vi "Monitor for Stop.vi"(7 "timeout":i32=200, 8 "error in (no error)":errorcluster, 9 "Mixed Mode Commands In":refnum<queue>, 11 "MM Button Events In":refnum<notifier>) -> (0 "error out":errorcluster, 1 "Mixed Mode Commands Out":refnum<queue>, 2 "Stop Requests":T1, 3 "Button Events Out":refnum<notifier>)   [LabVIEW 2009]
uses:
  MixedMode/Messages/Mixed Mode Button Events Message.ctl
  MixedMode/Messages/Mixed Mode Button Events.ctl
  Mixed Mode Widget Button States.ctl
  MixedMode/Messages/Mixed Mode Command.ctl
  MixedMode/Mixed Mode Command Action.ctl
  MixedMode/Ramp Time Tuple.ctl
  MixedMode/Target Data.ctl
  Stop Requests.ctl
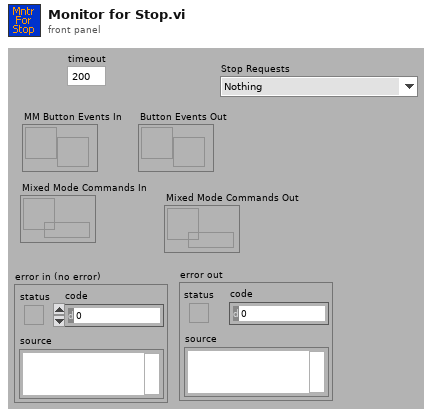
[diagram p1: front panel]
types:
  T1 = typedef "Stop Requests.ctl" = enum16{"Nothing", "Stop Requested", "Abort Requested"}
  T2 = typedef "Mixed Mode Command.ctl" = cluster{"Command":T3, "Ramp Times":cluster{"Initial":T4, "Iterative":T4}, "LBCB1":T5, "LBCB2":T5}
  T3 = typedef "Mixed Mode Command Action.ctl" = enum16{"Start Command", "Stop", "Exit", "No Op", "Start Acquisition", "Measure Initial Position"}
  T4 = typedef "Ramp Time Tuple.ctl" = cluster{"Ramp":dbl, "Stab":dbl, "Hold":dbl}
  T5 = typedef "Target Data.ctl" = cluster{"Displacements":dbl[], "Command Type":enum16{"<None>", "Displacement", "Force"}[], "Forces":dbl[]}
  T6 = typedef "Mixed Mode Button Events Message.ctl" = cluster{"MM Control Events":T7, "Button States":T8}
  T7 = typedef "Mixed Mode Button Events.ctl" = enum16{"Propose.Accept", "Propose.Decline", "Execute.Start", "Execute.Stop", "TargetSet", "InputFile.Load", "InputFile.Reset", "InputFile.Pause", "InputFile.Run", "CartesianType.Changed", "NCTP.ConnectToServer", "NTCP.DisconnectFromServer", "Application.Stop", "Control.Enabled", "Control.Disabled", "ControlType.Changed", "Nop", "Manual.SetInitialPosition"}
  T8 = typedef "Mixed Mode Widget Button States.ctl" = cluster{"Auto-Start Enabled":bool, "Auto-Accept Enabled":bool, "Exit Requested":bool, "Input File Loaded":bool, "Input File Running":bool, "NTCP Server  On":bool}
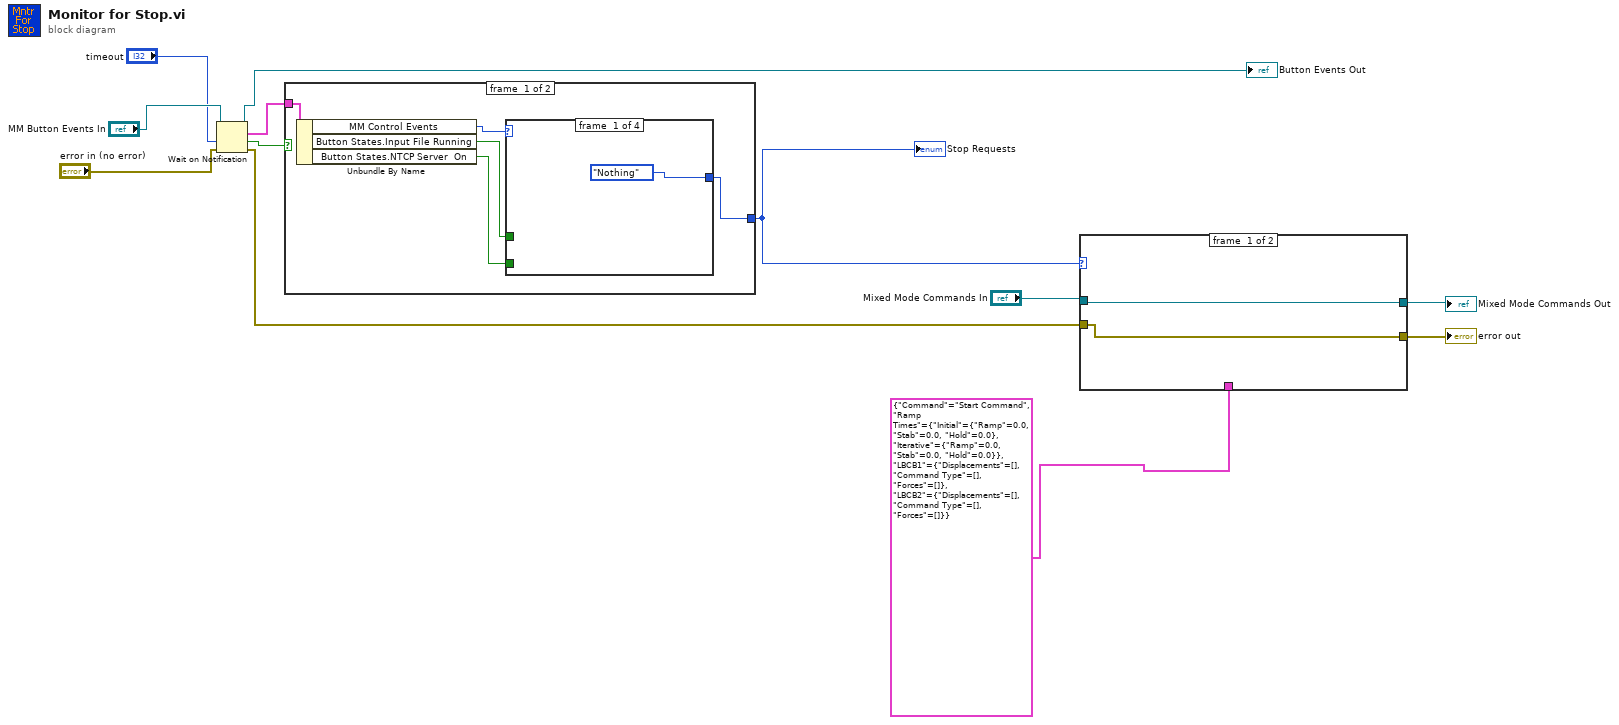
[diagram p0: block diagram]
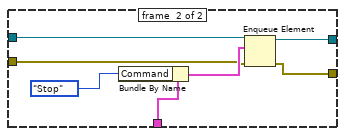
[diagram p2: hidden frame]
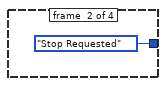
[diagram p3: hidden frame]
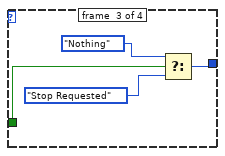
[diagram p4: hidden frame]
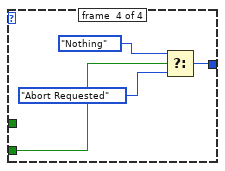
[diagram p5: hidden frame]
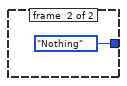
[diagram p6: hidden frame]
diagram:
  n1 = Wait on Notification(notifier="MM Button Events In", timeout in ms (-1)="timeout", error in (no error)="error in (no error)") -> (notifier out=→"Button Events Out":refnum<notifier>, notification=w7:T6, timed out?=w8:bool, error out=w5:errorcluster)  [unwired: 1 in]
  n2 = case shown="False" w8 {
    tunnel: w7 -> [w17 _]
    tunnel: [w15 Stop_Requests."Nothing" ("Stop Requested")] -> w1
    frame #0 {
      n3 = Unbundle By Name(w17) -> ("MM Control Events"=w16:T7, "Button States.Input File Running"=w14:bool, "Button States.NTCP Server  On"=w13:bool)
      n4 = case shown="\"Execute.Stop\"" w16 {
        tunnel: [Stop_Requests."Nothing" ("Stop Requested") Stop_Requests."Stop Requested" ("Stop Requested") w23 w26] -> w15
        tunnel: w14 -> [_ _ w21 _]
        tunnel: w13 -> [_ _ _ w25]
        frame #0 {
        }
        frame #1 {
        }
        frame #2 {
          n5 = Select(t=Stop_Requests."Nothing", s=w21, f=Stop_Requests."Stop Requested" ("Stop Requested")) -> (s? t:f=w23:T1)
        }
        frame #3 {
          n6 = Select(t=Stop_Requests."Nothing", s=w25, f=Stop_Requests."Abort Requested" ("Stop Requested")) -> (s? t:f=w26:T1)
        }
      }
    }
    frame #1 {
    }
  }
  "Stop Requests" <- w1
  n7 = case shown="\"Stop Requested\", Default" w1 {
    tunnel: "Mixed Mode Commands In" -> [w29 w37]
    tunnel: T2 {"Command"=enum."Start Command", "Ramp Times"={"Initial"={"Ramp"=0.0, "Stab"=0.0, "Hold"=0.0}, "Iterative"={"Ramp"=0.0, "Stab"=0.0, "Hold"=0.0}}, "LBCB1"={"Displacements"=[], "Command Type"=[], "Forces"=[]}, "LBCB2"={"Displacements"=[], "Command Type"=[], "Forces"=[]}} ("Mixed Mode Command") -> [_ w36]
    tunnel: [w29 w34] -> w2
    tunnel: [w30 w33] -> w6
    tunnel: w5 -> [w30 w32]
    frame #0 {
    }
    frame #1 {
      n8 = Bundle By Name(cluster=w36, "Command"=Mixed_Mode_Command_Action."Stop") -> (w35:T2)
      n9 = Enqueue Element(queue=w37, element=w35, error in (no error)=w32) -> (queue out=w34:refnum<queue>, error out=w33:errorcluster)  [unwired: 1 in, 1 out]
    }
  }
  "error out" <- w6
  "Mixed Mode Commands Out" <- w2
